vi "ingresaMediciones.vi"(8 "error in (no error)":errorcluster, 9 "Tbl Refnum":refnum<vi>, 10 "New Value":string[][](array[string]), 11 "Prueba09 in":refnum<class "Prueba10.lvclass">) -> (0 "error out":errorcluster, 3 "Prueba09 out":refnum<class "Prueba10.lvclass">)   [LabVIEW 2019, in "Prueba10.lvclass"]
uses:
  Prueba10.lvclass
  Prueba10.lvclass/Prueba10.ctl
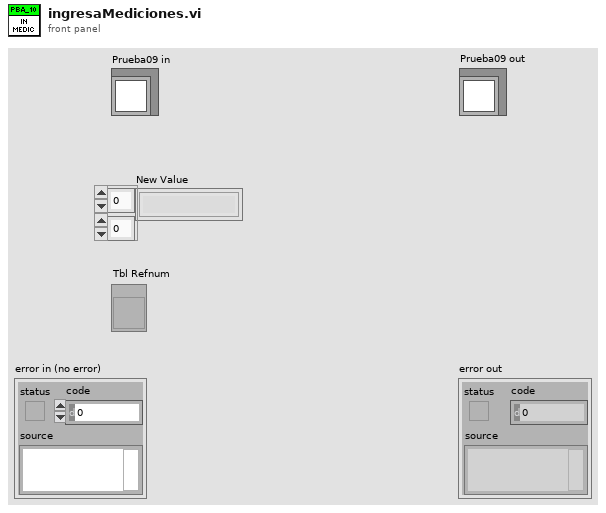
[diagram p1: front panel]
types:
  T1 = cluster{"Medido":dbl, "Error":dbl, "Ref":dbl, "Incert_exp":dbl, "Tol+":dbl, "Tol-":dbl, "fila":i32}
  T2 = typedef "LVRowAndColumnTypeDef.ctl" = cluster{"Row":i32, "Column":i32}
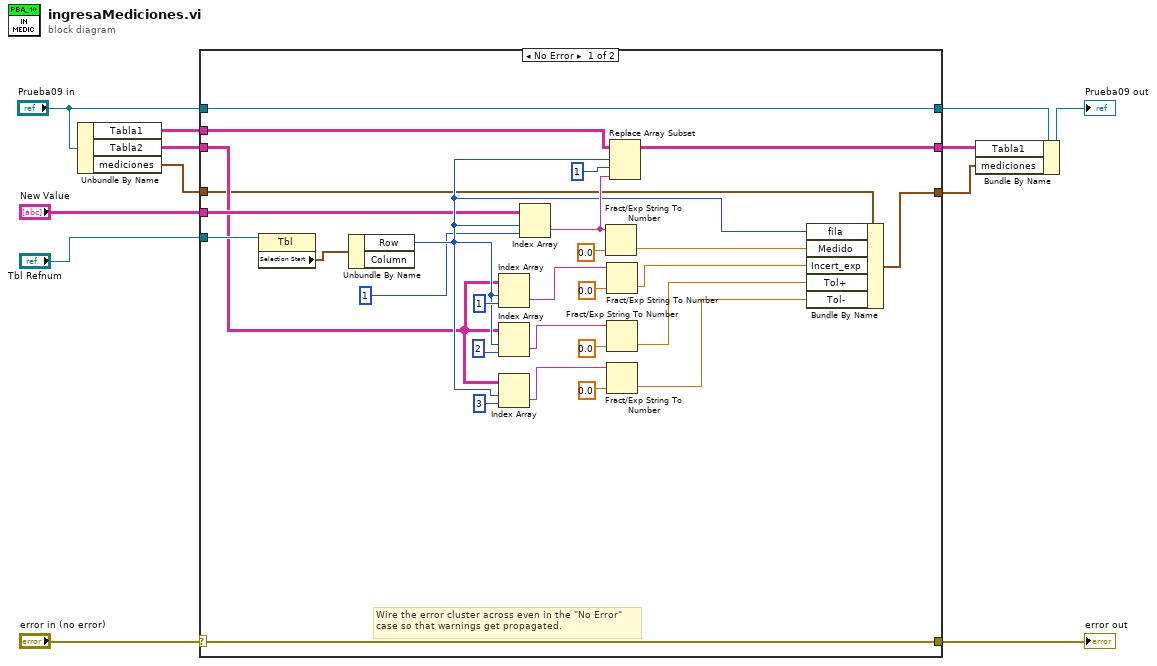
[diagram p0: block diagram]
diagram:
  n1 = Unbundle By Name("Prueba09 in") -> ("Tabla1"=w1:string[][], "Tabla2"=w6:string[][], "mediciones"=w5:T1)
  n2 = case shown="No Error" "error in (no error)" {
    selector: "error in (no error)" -> [w39 w44]
    tunnel: [w39 w44] -> w11
    tunnel: [w40 w43] -> w10
    tunnel: "Prueba09 in" -> [w40 w43]
    tunnel: w6 -> [w22 w42]
    tunnel: "New Value" -> [w25 _]
    tunnel: "Tbl Refnum" -> [w24 _]
    tunnel: w5 -> [w21 w41]
    tunnel: [w20 w42] -> w3
    tunnel: [w19 w41] -> w2
    tunnel: w1 -> [w17 _]
    frame No Error {
      # "Wire the error cluster across even in the \"No Error\"\ncase so that warnings get propagated."
      n3 = property on="Property Node" class="Tbl"(reference=w24) -> ("Selection Start"=w23:T2)  [unwired: 1 in, 2 out]
      n4 = Unbundle By Name(w23) -> ("Row"=w26:i32)  [unwired: 1 out]
      n5 = Index Array(array=w22, index (row)=w26, index (col)=1 ("disabled index (col)")) -> (element=w35:string)
      n6 = Index Array(array=w22, index (row)=w26, index (col)=2 ("index (row)")) -> (element=w31:string)
      n7 = Index Array(array=w22, index (row)=w26, index (col)=3 ("disabled index (col)")) -> (element=w28:string)
      n8 = Index Array(array=w25, index (row)=w26, index (col)=1 ("disabled index (col)")) -> (element=w27:string)
      n9 = Fract/Exp String To Number(string=w27, default (0 dbl)=0.0) -> (number=w18:dbl)  [unwired: 2 in, 1 out]
      n10 = Fract/Exp String To Number(string=w35, default (0 dbl)=0.0) -> (number=w16:dbl)  [unwired: 2 in, 1 out]
      n11 = Fract/Exp String To Number(string=w31, default (0 dbl)=0.0) -> (number=w15:dbl)  [unwired: 2 in, 1 out]
      n12 = Fract/Exp String To Number(string=w28, default (0 dbl)=0.0) -> (number=w14:dbl)  [unwired: 2 in, 1 out]
      n13 = Replace Array Subset(array=w17, new element=w27, index (row)=w26, index (col)=1 ("disabled index (col)")) -> (w20:string[][])
      n14 = Bundle By Name(cluster=w21, "fila"=w26, "Medido"=w18, "Incert_exp"=w16, "Tol+"=w15, "Tol-"=w14) -> (w19:T1)
    }
    frame Error {
    }
  }
  "error out" <- w11
  n15 = Bundle By Name(cluster=w10, "Tabla1"=w3, "mediciones"=w2) -> (→"Prueba09 out":refnum<class "Prueba10.lvclass">)
